vi "ABR3-Find Next Level.vi"(0 "Runtime":T1={"Ceiling"=0.0, "Threshold"=0.0, "Crossed?"=FALSE, "Step"=0, "Stop"=0, "Avgs"=0, "Level"=0.0, "AI Npts"=0, "Doubled?"=FALSE, "Gain"=0.0, "NWindowPts"=0, "dt"=0.0, "Cal"=path "", "Freq"=0.0, "AO Channels"=[], "AltPol"=FALSE, "AO Npts"=0, "AO Fs"=0.0, "Start"=0, "Stop max"=0, "Ear"=enum."Right", "Waveform"=enum."TONE PIP", "RepRate"=0.0, "CAP or ABR"=1, "LMasker"=0.0, "SeqVar"=enum."Signal Level", "Reps/buffer"=0, "Avg Mode"=enum."Neural/CM", "Wav"=path "", "Order"=enum."Sequential", "Levels"=[], "ControlVal"=0.0, "innerIndex"=0, "indexStep"=0} {"CAP or ABR" items=["CAP", "ABR"]}, 11 "error in (no error)":errorcluster) -> (4 "Runtime out":T1={"Ceiling"=0.0, "Threshold"=0.0, "Crossed?"=FALSE, "Step"=0, "Stop"=0, "Avgs"=0, "Level"=0.0, "AI Npts"=0, "Doubled?"=FALSE, "Gain"=0.0, "NWindowPts"=0, "dt"=0.0, "Cal"=path "", "Freq"=0.0, "AO Channels"=[], "AltPol"=FALSE, "AO Npts"=0, "AO Fs"=0.0, "Start"=0, "Stop max"=0, "Ear"=enum."Right", "Waveform"=enum."TONE PIP", "RepRate"=0.0, "CAP or ABR"=1, "LMasker"=0.0, "SeqVar"=enum."Signal Level", "Reps/buffer"=0, "Avg Mode"=enum."Neural/CM", "Wav"=path "", "Order"=enum."Sequential", "Levels"=[], "ControlVal"=0.0, "innerIndex"=0, "indexStep"=0} {"CAP or ABR" items=["CAP", "ABR"]}, 14 "Finished":bool, 15 "error out":errorcluster)   [LabVIEW 2020]
uses:
  TypeDefs/ABR3-Runtime Data.ctl
  epl-vi-lib/Utility VIs/Type Defs/Left-Right ring.ctl
  TypeDefs/ABR-Waveform Enum.ctl
  TypeDefs/ABR3-Seq Var Enum.ctl
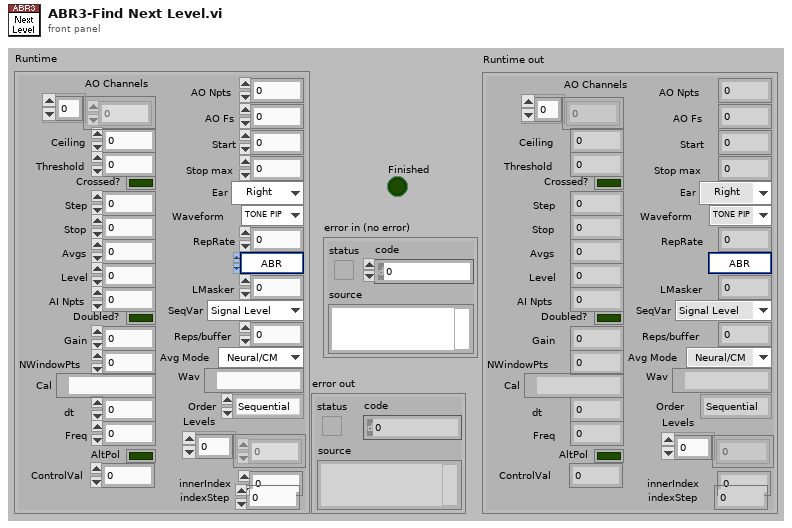
[diagram p1: front panel]
types:
  T1 = typedef "ABR3-Runtime Data.ctl" = cluster{"Ceiling":dbl, "Threshold":dbl, "Crossed?":bool, "Step":i32, "Stop":i32, "Avgs":i32, "Level":dbl, "AI Npts":i32, "Doubled?":bool, "Gain":dbl, "NWindowPts":i32, "dt":dbl, "Cal":path, "Freq":dbl, "AO Channels":i32[], "AltPol":bool, "AO Npts":i32, "AO Fs":dbl, "Start":i32, "Stop max":i32, "Ear":T2, "Waveform":T3, "RepRate":dbl, "CAP or ABR":u16, "LMasker":dbl, "SeqVar":T4, "Reps/buffer":i32, "Avg Mode":enum16{"Neural/CM", "ANOW"}, "Wav":path, "Order":enum16{"Sequential", "Random"}, "Levels":dbl[], "ControlVal":dbl, "innerIndex":i32, "indexStep":i32}
  T2 = typedef "Left-Right ring.ctl" = enum16{"Right", "Left"}
  T3 = typedef "ABR-Waveform Enum.ctl" = enum16{"TONE PIP", "CLICK", "FILE", "CHIRP", "NOISE", "VERHULST"}
  T4 = typedef "ABR3-Seq Var Enum.ctl" = enum16{"Signal Level", "Masker Level"}
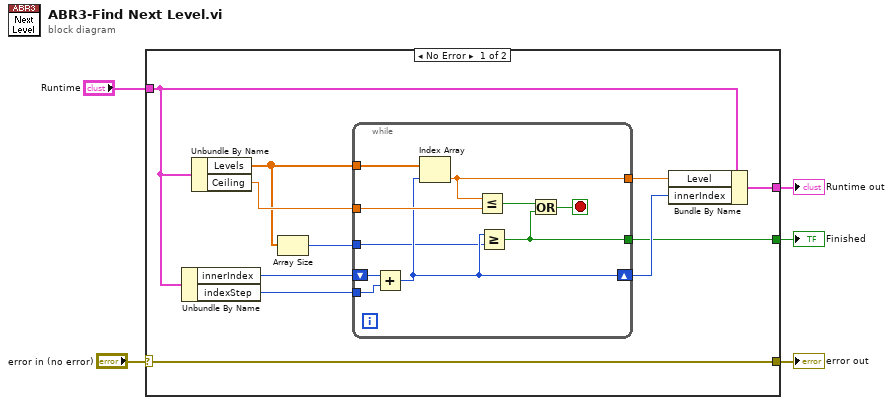
[diagram p0: block diagram]
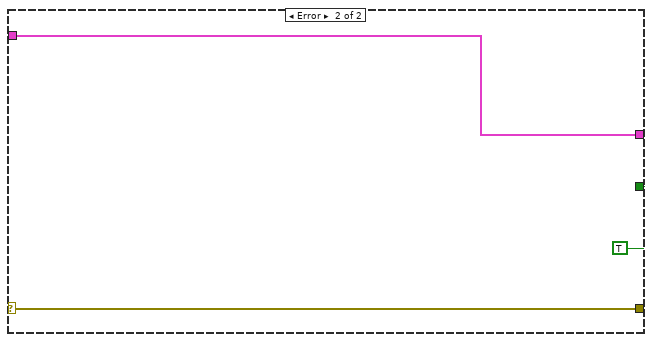
[diagram p2: hidden frame]
diagram:
  n1 = case shown="No Error" "error in (no error)" {
    selector: "error in (no error)" -> [w16 w28]
    tunnel: "Runtime" -> [w11 w29]
    tunnel: [w8 TRUE] -> w1
    tunnel: [w7 w29] -> w3
    tunnel: [w16 w28] -> w2
    frame No Error {
      n2 = Unbundle By Name(w11) -> ("innerIndex"=w15:i32, "indexStep"=w6:i32)
      n3 = Unbundle By Name(w11) -> ("Levels"=w13:dbl[], "Ceiling"=w14:dbl)
      n4 = Array Size(array=w13) -> (size(s)=w12:i32)
      n5 = while {
        tunnel: w13 -> [w26]
        shift-right: [w23] -> w9
        shift-left: w15 -> [w25]
        tunnel: w14 -> [w24]
        tunnel: w12 -> [w22]
        tunnel: [w19] -> w8
        tunnel: [w18] -> w10
        tunnel: w6 -> [w17]
        stop <- w20 stop-if-true
        n6 = Add(x=w25, y=w17) -> (x+y=w23:i32)
        n7 = Index Array(array=w26, index=w23) -> (element=w18:dbl)
        n8 = Less Or Equal?(x=w18, y=w24) -> (x <= y?=w21:bool)
        n9 = Greater Or Equal?(x=w23, y=w22) -> (x >= y?=w19:bool)
        n10 = Or(x=w21, y=w19) -> (x .or. y?=w20:bool)
      }
      n11 = Bundle By Name(cluster=w11, "Level"=w10, "innerIndex"=w9) -> (w7:T1)
    }
    frame Error {
    }
  }
  "error out" <- w2
  "Runtime out" <- w3
  "Finished" <- w1
